vi "input_pos.vi"(3 "error in (no error)":errorcluster, 4 "positie":dbl, 5 "VISA in":refnum<visa-resource-name>) -> (0 "error out":errorcluster, 2 "VISA out":refnum<visa-resource-name>)   [LabVIEW 2019]
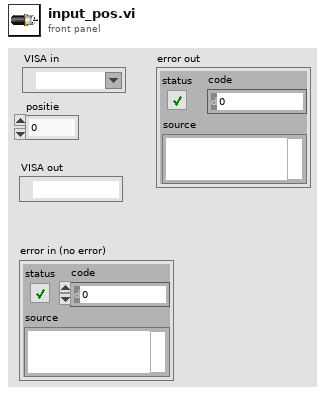
[diagram p1: front panel]
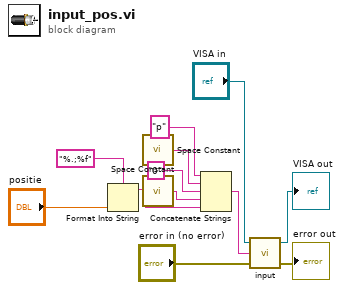
[diagram p0: block diagram]
diagram:
  n1 = Format Into String(format string="%.;%f", "positie") -> (resulting string=w5:string)  [unwired: 2 in, 1 out]
  n2 = call <vilib>:"Space Constant.vi"() -> ("String"=w10:string)
  n3 = call <vilib>:"Space Constant.vi"() -> ("String"=w12:string)
  n4 = Concatenate Strings("p" ("write buffer"), w10, "0", w12, w5) -> (w8:string)
  n5 = call "input.vi"("error in (no error)"="error in (no error)", "commando"=w8, "VISA in"="VISA in") -> ("error out"=→"error out":errorcluster, "VISA out"=→"VISA out":refnum<visa-resource-name>)  [unwired: 1 out]
